vi "Get Shift Values (Centroid).vi"(8 "error in (no error)":errorcluster, 11 "AVI Path":path) -> (0 "error out":errorcluster)   [LabVIEW 2012]
uses:
  <vilib>/vision/NI_Vision_Development_Module.lvlib
panel:
  out "Array":T1[](array[plugin-control])
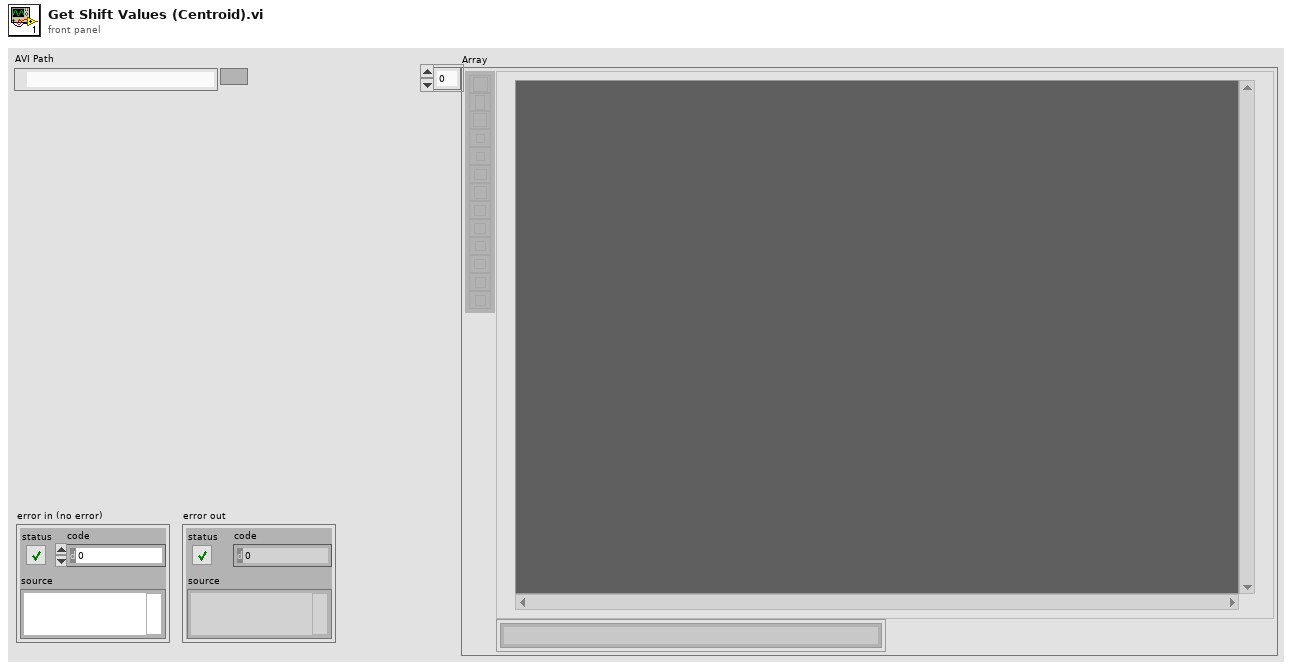
[diagram p1: front panel]
types:
  T1 = typedef "IMAQ Image.ctl" = refnum<image>
  T2 = cluster{"Position":cluster{"x":sgl, "y":sgl}, "Angle":sgl, "Scale":sgl, "Score":sgl, "Bounding Box":cluster{"x":sgl, "y":sgl}[]}[]
  T3 = cluster{"Position":cluster{"x":sgl, "y":sgl}, "Angle":sgl, "Scale":sgl, "Score":sgl, "Bounding Box":cluster{"x":sgl, "y":sgl}[]}
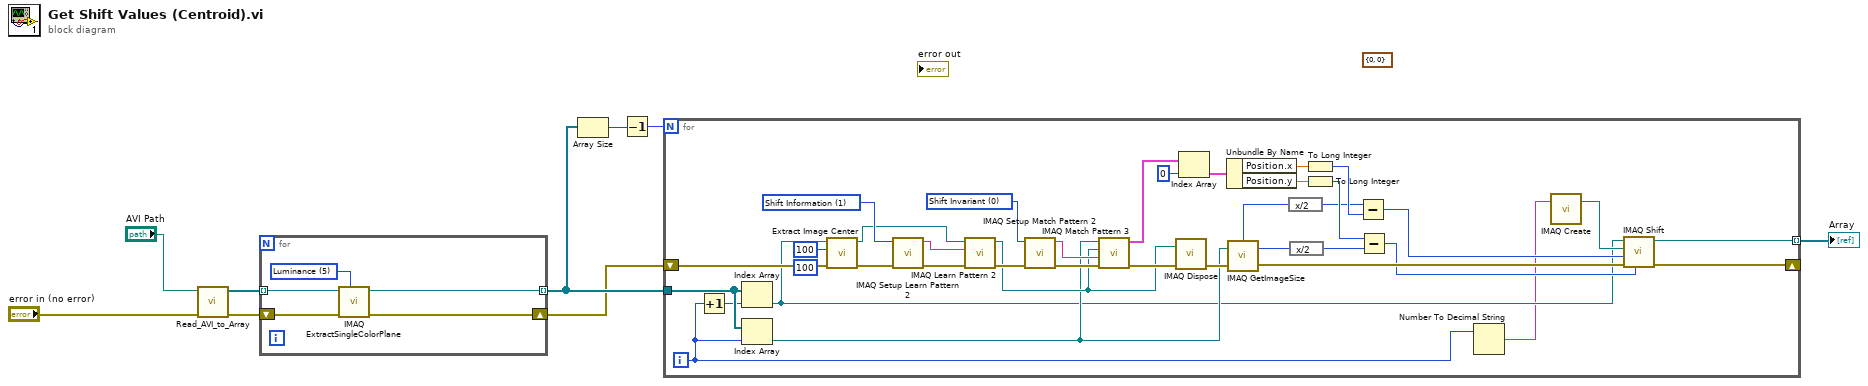
[diagram p0: block diagram]
diagram:
  (unwired) cluster{"dx":i32, "dy":i32} {"dx"=0, "dy"=0} ("Cluster")
  n1 = call "Read_AVI_to_Array.vi"("Error in (no error)"="error in (no error)", "AVI Path"="AVI Path") -> ("Error out"=w6:errorcluster, "Image Array"=w7:T1[])  [unwired: 7 in, 1 out]
  n2 = for {
    tunnel: w7 -> [w14] mode=indexing
    shift-right: [w12] -> w2
    shift-left: w6 -> [w13]
    tunnel: [w10] -> w5 mode=indexing
    w11 = 5 items=["Red", "Green", "Blue", "Hue", "Saturation", "Luminance", "Value", "Intensity"] ("Color Plane")
    n3 = call "IMAQ ExtractSingleColorPlane"("Color Plane"=w11, "error in (no error)"=w13, "Image Src"=w14) -> ("error out"=w12:errorcluster, "Image Dst Out"=w10:T1)  [unwired: 7 in]
  }
  n4 = Array Size(array=w5) -> (size(s)=w4:i32)
  n5 = Decrement(x=w4) -> (x-1=w3:i32)
  n6 = for {
    N: w3 -> [_]
    tunnel: w5 -> [w52]
    shift-right: [w22] -> _
    shift-left: w2 -> [w50]
    tunnel: [w18] -> w1 mode=indexing
    i -> [w17]
    w39 = u16 0 items=["Shift Invariant", "Rotation Invariant"] ("Match Mode")
    w45 = u16 1 items=["All", "Shift Information", "Rotation Information"] ("Learn Mode")
    n7 = Increment(x=w17) -> (x+1=w51:i32)
    n8 = Index Array(array=w52, index=w51) -> (element=w16:T1)
    n9 = Index Array(array=w52, index=w17) -> (element=w33:T1)
    n10 = call "Extract Image Center.vi"("error in (no error)"=w50, "y"=i64 100, "x"=i64 100, "Image"=w16) -> ("error out"=w44:errorcluster, "Image out"=w43:T1)  [unwired: 6 in]
    n11 = call "IMAQ Setup Learn Pattern 2"("error in (no error)"=w44, "Learn Mode"=w45) -> ("error out"=w47:errorcluster, "Learn Pattern Setup Data"=w46:string)  [unwired: 8 in]
    n12 = call "IMAQ Learn Pattern 2"("error in (no error)"=w47, "Learn Pattern Setup Data"=w46, "Image"=w43) -> ("error out"=w42:errorcluster, "Template Image Out"=w35:T1)  [unwired: 7 in]
    n13 = call "IMAQ Setup Match Pattern 2"("error in (no error)"=w42, "Match Mode"=w39) -> ("error out"=w41:errorcluster, "Match Pattern Setup Data"=w40:string)  [unwired: 8 in]
    n14 = call "IMAQ Match Pattern 3"("error in (no error)"=w41, "Match Pattern Setup Data"=w40, "Template Image"=w35, "Image"=w33) -> ("error out"=w36:errorcluster, "Matches"=w38:T2)  [unwired: 5 in, 1 out]
    n15 = call "IMAQ Dispose"("Image"=w35, "error in (no error)"=w36) -> ("error out"=w34:errorcluster)  [unwired: 4 in]
    n16 = Index Array(array=w38, index=0) -> (element=w37:T3)
    n17 = Unbundle By Name(w37) -> ("Position.x"=w32:sgl, "Position.y"=w31:sgl)
    n18 = call "IMAQ GetImageSize"("Image"=w33, "error in (no error)"=w34) -> ("Y Resolution"=w26:i32, "X Resolution"=w28:i32, "error out"=w23:errorcluster)  [unwired: 2 in]
    n19 = expression code="x/2"(w28) -> (w27:i32)
    n20 = expression code="x/2"(w26) -> (w25:i32)
    n21 = To Long Integer(number=w32) -> (32bit integer=w30:i32)
    n22 = To Long Integer(number=w31) -> (32bit integer=w29:i32)
    n23 = Subtract(x=w27, y=w30) -> (x-y=w21:i32)
    n24 = Subtract(x=w29, y=w25) -> (x-y=w20:i32)
    n25 = Number To Decimal String(number=w17) -> (decimal integer string=w15:string)  [unwired: 1 in]
    n26 = call "IMAQ Create"("Image Name"=w15) -> ("New Image"=w19:T1)  [unwired: 4 in, 1 out]
    n27 = call "IMAQ Shift"("YOffset"=w20, "error in (no error)"=w23, "XOffset"=w21, "Image Dst"=w19, "Image Src"=w16) -> ("error out"=w22:errorcluster, "Image Dst Out"=w18:T1)  [unwired: 5 in]
  }
  "Array" <- w1
